vi "aal_CIC.vi"   [LabVIEW 2020, in "NI_AALPro.lvlib"]
uses:
  NI_AALPro.lvlib
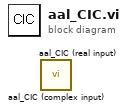
[diagram p0: block diagram]
diagram:
  n1 = call "aal_CIC (complex input).vi"() -> ()  [unwired: 4 in, 1 out]
  n2 = call "aal_CIC (real input).vi"() -> ()  [unwired: 4 in, 1 out]
